vi "Apply EL Mode.vi"(8 "error in (no error)":errorcluster, 11 "Motor in":refnum<class "Motor.lvclass">) -> (0 "error out":errorcluster, 3 "Motor out":refnum<class "Motor.lvclass">)   [LabVIEW 2016, in "Hardware.lvlib" / "Motor.lvlib" / "Motor.lvclass"]
uses:
  <userlib>/Common Components/Hardware/Motor/Motor/Motor.lvclass
  <userlib>/Common Components/Hardware/Motor/Motor/Motor.lvclass/Motor.ctl
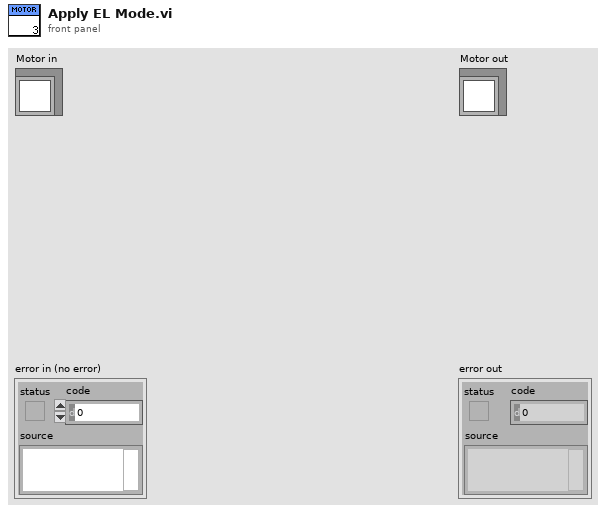
[diagram p1: front panel]
types:
  T1 = enum16{"both +- disabled", "both +- enabled", "+ disabled, - enabled", "+ enabled, - disabled"}
  T2 = enum16{"both +- stop immediately", "both +- decelerate to stop", "+ stop immediately, - decelerate to stop", "+ decelerate to stop, - stop immediately"}
  T3 = enum16{"both +- logical low", "both +- logical high", "+ logical low, - logical high", "+ logical high, - logical low"}
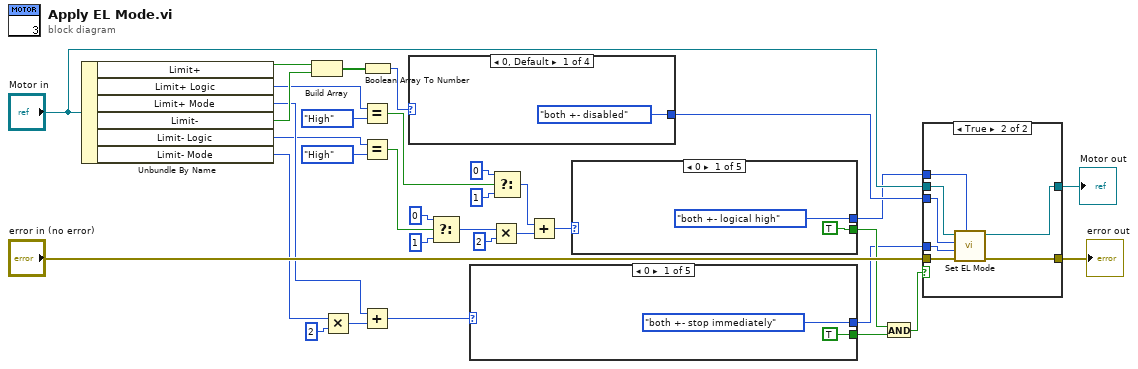
[diagram p0: block diagram]
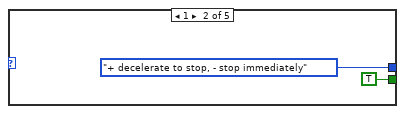
[diagram p2: hidden frame]
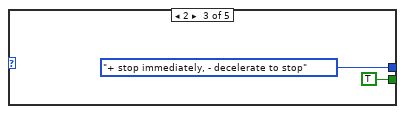
[diagram p3: hidden frame]
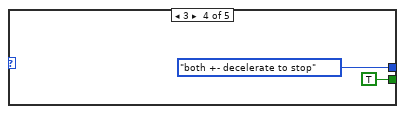
[diagram p4: hidden frame]
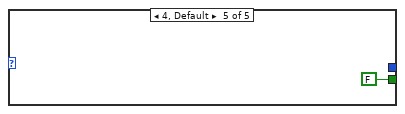
[diagram p5: hidden frame]
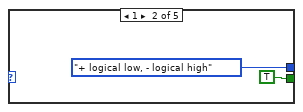
[diagram p7: hidden frame]
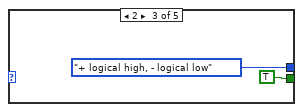
[diagram p8: hidden frame]
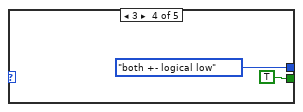
[diagram p9: hidden frame]
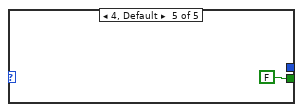
[diagram p10: hidden frame]
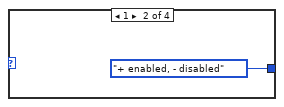
[diagram p11: hidden frame]
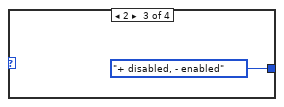
[diagram p12: hidden frame]
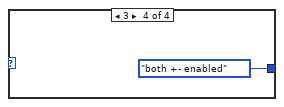
[diagram p13: hidden frame]
diagram:
  n1 = Unbundle By Name("Motor in") -> ("Limit+"=w29:bool, "Limit+ Logic"=w12:enum16{"Low", "High"}, "Limit+ Mode"=w17:enum16{"Stop immediately", "Decelerate to Stop"}, "Limit-"=w28:bool, "Limit- Logic"=w2:enum16{"Low", "High"}, "Limit- Mode"=w16:enum16{"Stop immediately", "Decelerate to Stop"})
  n2 = Build Array(w29, w28) -> (w30:bool[])
  n3 = Multiply(x=w16, y=2) -> (x*y=w19:i32)
  n4 = Equal?(x=w12, y=enum16{"Low", "High"}."High") -> (x = y?=w11:bool)
  n5 = Equal?(x=w2, y=enum16{"Low", "High"}."High") -> (x = y?=w3:bool)
  n6 = Add(x=w17, y=w19) -> (x+y=w18:i32)
  n7 = Boolean Array To Number(Boolean array=w30) -> (number=w27:u32)
  n8 = case shown="0, Default" w27 {
    tunnel: [T1."both +- disabled" ("el_enableEL") T1."+ enabled, - disabled" ("el_enableEL") T1."+ disabled, - enabled" ("el_enableEL") T1."both +- enabled" ("el_enableEL")] -> w26
    frame 0, Default {
    }
    frame 1 {
    }
    frame 2 {
    }
    frame 3 {
    }
  }
  n9 = Select(t=0, s=w3, f=1) -> (s? t:f=w1:i32)
  n10 = case shown="0" w18 {
    tunnel: [T2."both +- stop immediately" ("el_modeEL") T2."+ decelerate to stop, - stop immediately" ("el_modeEL") T2."+ stop immediately, - decelerate to stop" ("el_modeEL") T2."both +- decelerate to stop" ("el_modeEL") _] -> w15
    tunnel: [TRUE TRUE TRUE TRUE FALSE] -> w13
    frame 0 {
    }
    frame 1 {
    }
    frame 2 {
    }
    frame 3 {
    }
    frame 4, Default {
    }
  }
  n11 = Multiply(x=w1, y=2) -> (x*y=w24:i32)
  n12 = Select(t=0, s=w11, f=1) -> (s? t:f=w7:i32)
  n13 = Add(x=w7, y=w24) -> (x+y=w23:i32)
  n14 = case shown="0" w23 {
    tunnel: [T3."both +- logical high" ("el_logicEL") T3."+ logical low, - logical high" ("el_logicEL") T3."+ logical high, - logical low" ("el_logicEL") T3."both +- logical low" ("el_logicEL") _] -> w22
    tunnel: [TRUE TRUE TRUE TRUE FALSE] -> w21
    frame 0 {
    }
    frame 1 {
    }
    frame 2 {
    }
    frame 3 {
    }
    frame 4, Default {
    }
  }
  n15 = And(x=w21, y=w13) -> (x .and. y?=w14:bool)
  n16 = case shown="True" w14 {
    tunnel: "error in (no error)" -> [w57 w65]
    tunnel: [w57 w64] -> w33
    tunnel: [w58 w63] -> w32
    tunnel: "Motor in" -> [w58 w62]
    tunnel: w26 -> [_ w61]
    tunnel: w22 -> [_ w60]
    tunnel: w15 -> [_ w59]
    frame False {
    }
    frame True {
      n17 = call-dynamic "Set EL Mode.vi"("el_logicEL"=w60, "error in (no error)"=w65, "el_modeEL"=w59, "el_enableEL"=w61, "Motor in"=w62) -> ("error out"=w64:errorcluster, "Motor out"=w63:refnum<class "Motor.lvclass">)  [unwired: 5 in]
    }
  }
  "error out" <- w33
  "Motor out" <- w32
